vi "WritePolaration.vi"(1 "本次文件名":string) -> ()   [LabVIEW 2018]
uses:
  Init/AllPath.vi
  Reslut.vi
  <vilib>/Utility/file.llb/Write Delimited Spreadsheet (string).vi
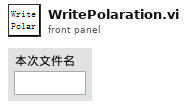
[diagram p1: front panel]
types:
  T1 = cluster{" 偏振方向":string, "偏振度":string, " 偏振方向 单位 ":string, "偏振度单位":string}
  T2 = cluster{"激光器型号":string, "X":dbl, "Y":dbl, "Z":dbl, "Rotate":dbl, "Pitching":dbl}
  T3 = cluster{"能量/功率":path, " 示波器":path, " 光谱仪":path, "偏振":path, "近远场":cluster{" 近场图片":path, " 远场图片":path, "发散角数据":path}, "参数":path, " 基路径":path, "文件名信息":path}
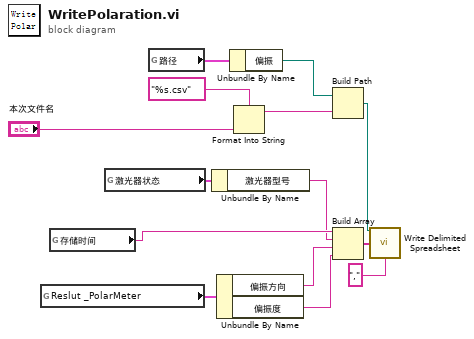
[diagram p0: block diagram]
diagram:
  n1 = global read "Reslut.vi" "Reslut _PolarMeter"() -> (w11:T1)
  n2 = global read "Reslut.vi" "存储时间"() -> (w2:string)
  n3 = global read "参数.vi" "激光器状态"() -> (w12:T2)
  n4 = global read "AllPath.vi" "路径"() -> (w14:T3)
  n5 = Unbundle By Name(w12) -> ("激光器型号"=w1:string)
  n6 = Unbundle By Name(w11) -> ("偏振方向"=w4:string, "偏振度"=w3:string)
  n7 = Unbundle By Name(w14) -> ("偏振"=w13:path)
  n8 = Format Into String(format string="%s.csv" ("格式字符串"), "本次文件名") -> (resulting string=w5:string)  [unwired: 2 in, 1 out]
  n9 = Build Path(base path=w13, name or relative path=w5) -> (appended path=w9:path)
  n10 = Build Array(w2, w1, w4, w3) -> (w10:string[])
  n11 = call-poly <vilib>:"Write Delimited Spreadsheet.vi"("file path (dialog if empty)"=w9, "1D data"=w10, "delimiter (\\t)"="," ("delimiter (\\t)")) -> ()  [unwired: 11 in, 2 out]
